vi "Random_2D_Array.vi"() -> ()   [LabVIEW 2022 SP3]
panel:
  out "Random 5x10":dbl[][](array[numeric])
  # "Random_2D_Array:\nRun the program to create a random 2D array\nof dimensions 5x10."
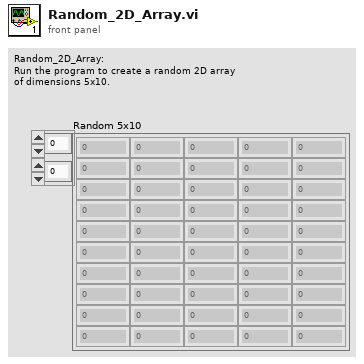
[diagram p1: front panel]
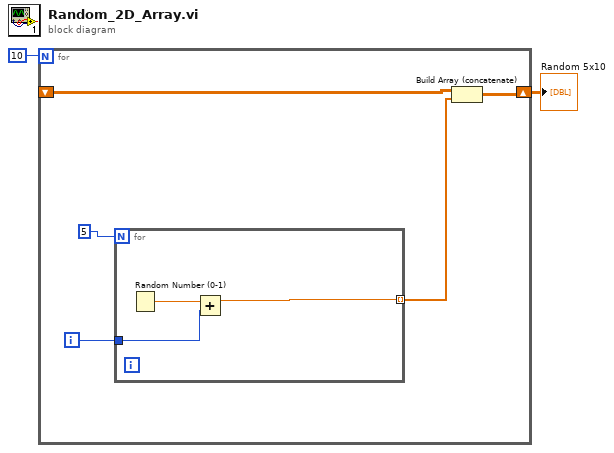
[diagram p0: block diagram]
diagram:
  n1 = for {
    N: 10 -> [_]
    shift-right: [w4] -> w1
    shift-left: _ -> [w5]
    i -> [w6]
    n2 = for {
      N: 5 -> [_]
      tunnel: [w9] -> w3 mode=indexing
      tunnel: w6 -> [w8]
      n3 = Random Number (0-1)() -> (number: 0 to 1=w10:dbl)
      n4 = Add(x=w10, y=w8) -> (x+y=w9:dbl)
    }
    n5 = Build Array (concatenate)(w5, w3) -> (w4:dbl[][])
  }
  "Random 5x10" <- w1
